vi "FrequencySet_Core_NB.vi"(0 "NB VCO Frequency":i32=2400, 5 "NB Did":i32 min=0 max=2 step=1, 7 "Core VCO Frequency":i32=2400, 9 "Core Did":i32 min=0 max=2 step=1, 11 "error in":errorcluster) -> (15 "error out":errorcluster)   [LabVIEW 2011]
doc: "This VI sets the frequency of the Core and NB PLL's.\n\nInputs:\n1. NB Frequency: Selects the frequency that the NB PLL will be set to.\n2. NB Did: The Did value of the NB frequency.\n3. Core Frequency: Selects the frequency that the Core PLL's will be set to.\n4. Core Did: The Did value of the Core frequency."
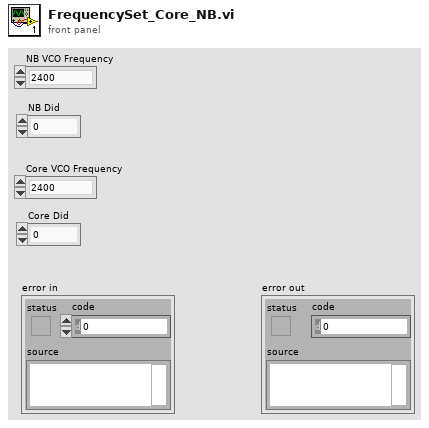
[diagram p1: front panel]
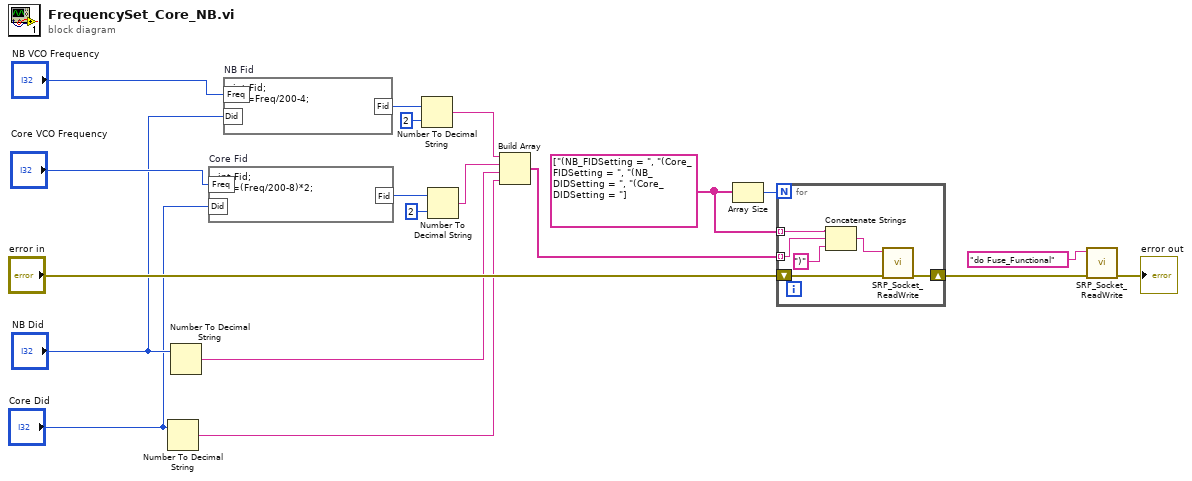
[diagram p0: block diagram]
diagram:
  w6 = string[] ["(NB_FIDSetting = ", "(Core_FIDSetting = ", "(NB_DIDSetting = ", "(Core_DIDSetting = "]
  n1 = Number To Decimal String(number="Core Did") -> (decimal integer string=w3:string)  [unwired: 1 in]
  n2 = Number To Decimal String(number="NB Did") -> (decimal integer string=w4:string)  [unwired: 1 in]
  n3 = formula code="int Fid;\nFid=(Freq/200-8)*2;" "Core Fid"("Freq"="Core VCO Frequency", "Did"="Core Did") -> ("Fid"=w12:i32)
  n4 = formula code="int Fid;\nFid=Freq/200-4;" "NB Fid"("Freq"="NB VCO Frequency", "Did"="NB Did") -> ("Fid"=w13:i32)
  n5 = Number To Decimal String(number=w13, width (-)=i16 2) -> (decimal integer string=w9:string)
  n6 = Number To Decimal String(number=w12, width (-)=i16 2) -> (decimal integer string=w8:string)
  n7 = Build Array(w9, w8, w4, w3) -> (w7:string[])
  n8 = Array Size(array=w6) -> (size(s)=w11:i32)
  n9 = for {
    N: w11 -> [_]
    tunnel: w6 -> [w24] mode=indexing
    shift-right: [w22] -> w10
    shift-left: "error in" -> [w23]
    tunnel: w7 -> [w21] mode=indexing
    n10 = Concatenate Strings(w24, w21, ")") -> (w20:string)
    n11 = call "SRP_Socket_ReadWrite.vi"("error in (no error)"=w23, "Data In"=w20) -> ("error out"=w22:errorcluster)  [unwired: 7 in, 1 out]
  }
  n12 = call "SRP_Socket_ReadWrite.vi"("error in (no error)"=w10, "Data In"="do Fuse_Functional") -> ("error out"=→"error out":errorcluster)  [unwired: 7 in, 1 out]
